vi "Initialise.vi"(4 "Rate (Hz)":dbl=1000.0 format="%0.2f", 6 "WarmupIters":u32=2000, 8 "error in (no error)":errorcluster, 9 "Master Clock":tag, 10 "Tasks Config":T1[](array[typedef]), 11 "PXI in":refnum<class "PXI.lvclass">) -> (0 "error out":errorcluster, 3 "PXI out":refnum<class "PXI.lvclass">)   [LabVIEW 2013, in "PXI.lvclass"]
uses:
  PXI.lvclass
  Task Definition.ctl
  Task Types.ctl
  PXI.lvclass/PXI.ctl
  <vilib>/DAQmx/create/channels.llb/DAQmx Create Channel (AI-Voltage-Basic).vi
  <vilib>/DAQmx/configure/timing.llb/DAQmx Timing (Sample Clock).vi
  <vilib>/DAQmx/create/channels.llb/DAQmx Create Channel (AO-Voltage-Basic).vi
  <vilib>/DAQmx/create/channels.llb/DAQmx Create Channel (DI-Digital Input).vi
  <vilib>/DAQmx/create/channels.llb/DAQmx Create Channel (DO-Digital Output).vi
  <resource>/objmgr/daqmx.rc
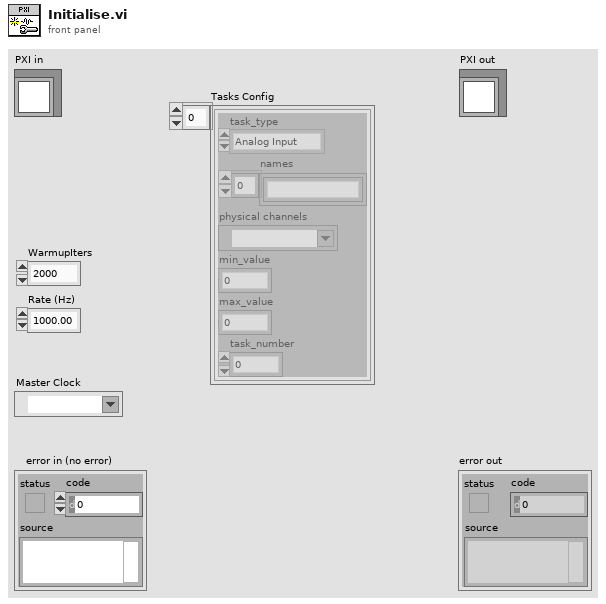
[diagram p1: front panel]
types:
  T1 = typedef "Task Definition.ctl" = cluster{"task_type":T2, "names":string[], "physical channels":tag, "min_value":dbl, "max_value":dbl, "task_number":i32}
  T2 = typedef "Task Types.ctl" = enum16{"Analog Input", "Analog Output", "Digital Input", "Digital Output"}
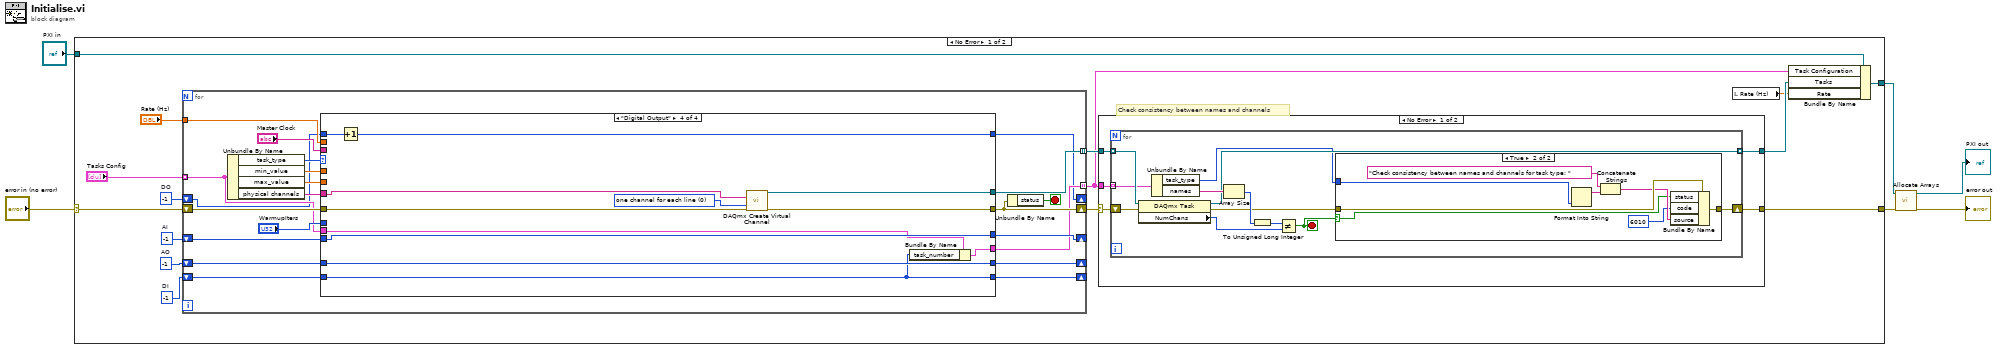
[diagram p0: block diagram]
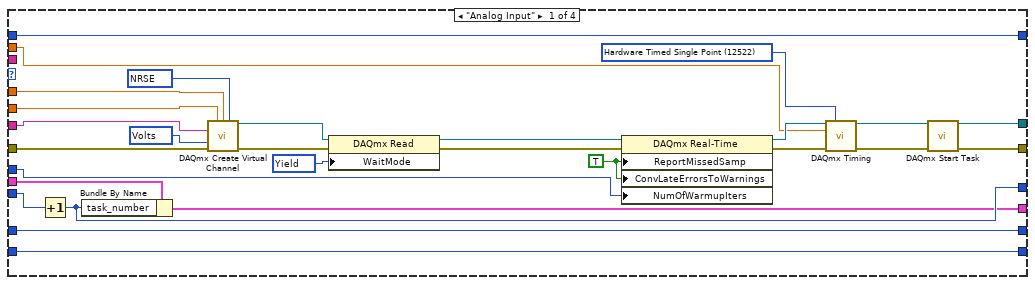
[diagram p4: hidden frame]
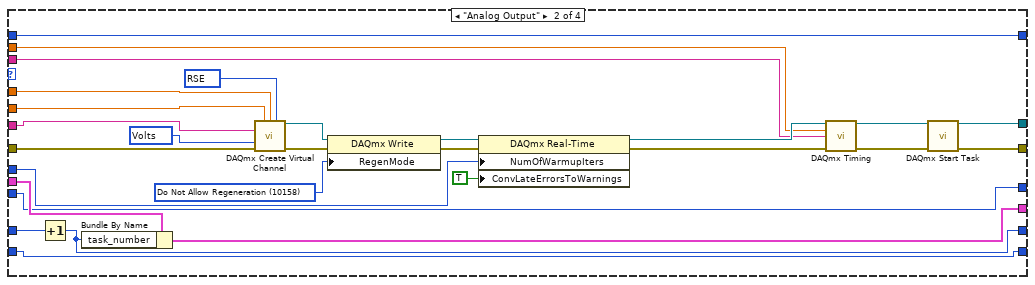
[diagram p5: hidden frame]
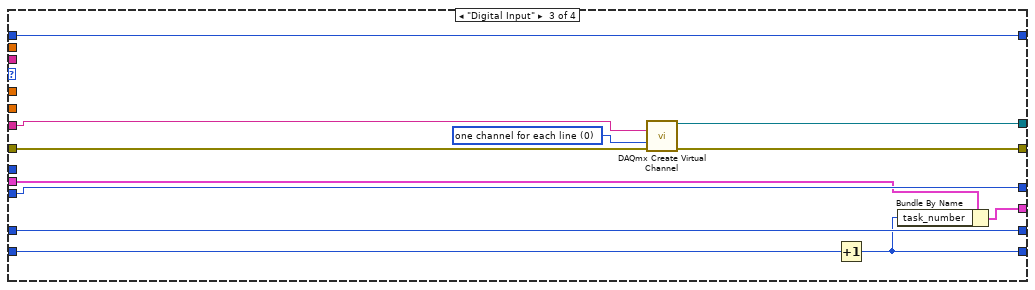
[diagram p6: hidden frame]
diagram:
  n1 = case shown="No Error" "error in (no error)" {
    selector: "error in (no error)" -> [w19 w152]
    tunnel: [w17 w152] -> w3
    tunnel: [w20 w151] -> w4
    tunnel: "PXI in" -> [w21 w151]
    frame No Error {
      w7 = -1  # DO
      w8 = -1  # DI
      w9 = -1  # AO
      w10 = -1  # AI
      # "Check consistency between names and channels"
      n2 = for {
        tunnel: "Tasks Config" -> [w58] mode=indexing
        tunnel: [w65] -> w16 mode=indexing
        shift-right: [w63] -> w18
        shift-left: w19 -> [w64]
        tunnel: "Rate (Hz)" -> [w60]
        tunnel: [w57] -> w11 mode=indexing
        shift-right: [w59] -> _
        shift-left: w10 -> [w56]
        shift-right: [w54] -> _
        shift-left: w9 -> [w55]
        shift-right: [w52] -> _
        shift-left: w8 -> [w53]
        shift-right: [w50] -> _
        shift-left: w7 -> [w51]
        stop <- w62 stop-if-true
        n3 = Unbundle By Name(w58) -> ("task_type"=w61:T2, "min_value"=w69:dbl, "max_value"=w68:dbl, "physical channels"=w67:tag)
        n4 = case shown="\"Digital Output\"" w61 {
          tunnel: w69 -> [w96 w113 _ _]
          tunnel: w68 -> [w95 w112 _ _]
          tunnel: w67 -> [w94 w106 w137 w149]
          tunnel: "WarmupIters" -> [w84 w116 _ _]
          tunnel: "Master Clock" -> [_ w115 _ _]
          tunnel: w60 -> [w83 w114 _ _]
          tunnel: [w80 w109 w136 w148] -> w65
          tunnel: [w79 w108 w135 w147] -> w63
          tunnel: w64 -> [w78 w107 w134 w146]
          tunnel: w56 -> [w77 w101 w133 w145]
          tunnel: [w75 w101 w133 w145] -> w59
          tunnel: w58 -> [w76 w104 w131 w142]
          tunnel: [w74 w103 w130 w143] -> w57
          tunnel: w55 -> [w73 w105 w132 w144]
          tunnel: [w73 w102 w132 w144] -> w54
          tunnel: w53 -> [w72 w100 w129 w139]
          tunnel: [w72 w100 w127 w139] -> w52
          tunnel: w51 -> [w71 w99 w128 w141]
          tunnel: [w71 w99 w128 w140] -> w50
          frame "Analog Input" {
            w85 = TRUE ("ConvLateErrorsToWarnings")
            w88 = 12522 items=["Finite Samples"=10178, "Continuous Samples"=10123, "Hardware Timed Single Point"=12522] ("sample mode")
            w93 = 12525 items=["Wait For Interrupt"=12523, "Poll"=12524, "Yield"=12525, "Sleep"=12547] ("WaitMode")
            w97 = 10348 items=["Volts"=10348, "From Custom Scale"=10065] ("units")
            w98 = 10078 items=["default"=-1, "RSE"=10083, "NRSE"=10078, "Differential"=10106, "Pseudodifferential"=12529] ("input terminal configuration")
            n5 = Increment(x=w77) -> (x+1=w75:i32)
            n6 = Bundle By Name(cluster=w76, "task_number"=w75) -> (w74:T1)
            n7 = call-poly <vilib>:"DAQmx Create Virtual Channel.vi"("maximum value"=w95, "minimum value"=w96, "input terminal configuration"=w98, "physical channels"=w94, "units"=w97, "error in"=w78) -> ("task out"=w87:refnum<k21>, "error out"=w86:errorcluster)  [unwired: 8 in]
            n8 = property class="DAQmx Read"(reference=w87, error in=w86, "WaitMode"=w93) -> (reference out=w91:refnum<k21>, error out=w92:errorcluster)
            n9 = property class="DAQmx Real-Time"(reference=w91, error in=w92, "ReportMissedSamp"=w85, "ConvLateErrorsToWarnings"=w85, "NumOfWarmupIters"=w84) -> (reference out=w89:refnum<k21>, error out=w90:errorcluster)
            n10 = call-poly <vilib>:"DAQmx Timing.vi"("task/channels in"=w89, "sample mode"=w88, "rate"=w83, "error in"=w90) -> ("task out"=w82:refnum<k21>, "error out"=w81:errorcluster)  [unwired: 10 in]
            n11 = call <vilib>:"DAQmx Start Task.vi"("task/channels in"=w82, "error in"=w81) -> ("task out"=w80:refnum<k21>, "error out"=w79:errorcluster)  [unwired: 12 in]
          }
          frame "Analog Output" {
            w123 = 10158 items=["Allow Regeneration"=10097, "Do Not Allow Regeneration"=10158] ("RegenMode")
            w126 = 10083 items=["Default"=-1, "RSE"=10083, "Differential"=10106, "Pseudodifferential"=12529] ("output terminal configuration")
            w125 = 10348 items=["Volts"=10348, "From Custom Scale"=10065] ("units")
            n12 = Increment(x=w105) -> (x+1=w102:i32)
            n13 = Bundle By Name(cluster=w104, "task_number"=w102) -> (w103:T1)
            n14 = call-poly <vilib>:"DAQmx Create Virtual Channel.vi"("maximum value"=w112, "minimum value"=w113, "output terminal configuration"=w126, "physical channels"=w106, "units"=w125, "error in"=w107) -> ("task out"=w122:refnum<k21>, "error out"=w121:errorcluster)  [unwired: 8 in]
            n15 = property class="DAQmx Write"(reference=w122, error in=w121, "RegenMode"=w123) -> (reference out=w120:refnum<k21>, error out=w119:errorcluster)
            n16 = property class="DAQmx Real-Time"(reference=w120, error in=w119, "NumOfWarmupIters"=w116, "ConvLateErrorsToWarnings"=TRUE ("ReportMissedSamp")) -> (reference out=w118:refnum<k21>, error out=w117:errorcluster)
            n17 = call-poly <vilib>:"DAQmx Timing.vi"("task/channels in"=w118, "rate"=w114, "source"=w115, "error in"=w117) -> ("task out"=w111:refnum<k21>, "error out"=w110:errorcluster)  [unwired: 10 in]
            n18 = call <vilib>:"DAQmx Start Task.vi"("task/channels in"=w111, "error in"=w110) -> ("task out"=w109:refnum<k21>, "error out"=w108:errorcluster)  [unwired: 12 in]
          }
          frame "Digital Input" {
            w138 = 0 items=["one channel for each line", "one channel for all lines"] ("line grouping")
            n19 = call-poly <vilib>:"DAQmx Create Virtual Channel.vi"("lines"=w137, "line grouping"=w138, "error in"=w134) -> ("task out"=w136:refnum<k21>, "error out"=w135:errorcluster)  [unwired: 11 in]
            n20 = Increment(x=w129) -> (x+1=w127:i32)
            n21 = Bundle By Name(cluster=w131, "task_number"=w127) -> (w130:T1)
          }
          frame "Digital Output" {
            w150 = 0 items=["one channel for each line", "one channel for all lines"] ("line grouping")
            n22 = Increment(x=w141) -> (x+1=w140:i32)
            n23 = call-poly <vilib>:"DAQmx Create Virtual Channel.vi"("lines"=w149, "line grouping"=w150, "error in"=w146) -> ("task out"=w148:refnum<k21>, "error out"=w147:errorcluster)  [unwired: 11 in]
            n24 = Bundle By Name(cluster=w142, "task_number"=w139) -> (w143:T1)
          }
        }
        n25 = Unbundle By Name(w63) -> ("status"=w62:bool)
      }
      n26 = case shown="No Error" w18 {
        selector: w18 -> [w24 w49]
        tunnel: [w22 w49] -> w17
        tunnel: w16 -> [w25 w48]
        tunnel: w11 -> [w26 _]
        tunnel: [w23 w48] -> w14
        frame No Error {
          n27 = for {
            tunnel: w26 -> [w36] mode=indexing
            tunnel: w25 -> [w38] mode=indexing
            tunnel: [w31] -> w23 mode=indexing
            shift-right: [w28] -> w22
            shift-left: w24 -> [w37]
            stop <- w30 stop-if-true
            n28 = property class="DAQmx Task"(reference=w38, error in=w37) -> (reference out=w31:refnum<k21>, error out=w29:errorcluster, "NumChans"=w34:u32)
            n29 = Unbundle By Name(w36) -> ("task_type"=w27:T2, "names"=w35:string[])
            n30 = Array Size(array=w35) -> (size(s)=w33:i32)
            n31 = To Unsigned Long Integer(number=w33) -> (unsigned 32bit integer=w32:u32)
            n32 = Not Equal?(x=w32, y=w34) -> (x != y?=w30:bool)
            n33 = case shown="True" w30 {
              selector: w30 -> [_ w40]
              tunnel: w29 -> [w39 w47]
              tunnel: [w39 w46] -> w28
              tunnel: w27 -> [_ w45]
              frame False {
              }
              frame True {
                n34 = Format Into String(w45) -> (resulting string=w44:string)  [unwired: 3 in, 1 out]
                n35 = Concatenate Strings("Check consistency between names and channels for task type: " ("source"), w44) -> (w42:string)
                n36 = Bundle By Name(cluster=w47, "status"=w40, "code"=6010, "source"=w42) -> (w46:errorcluster)
              }
            }
          }
        }
        frame Error {
        }
      }
      n37 = local read "Rate (Hz)"() -> (w12:dbl)
      n38 = Bundle By Name(cluster=w21, "Task Configuration"=w11, "Tasks"=w14, "Rate"=w12) -> (w20:refnum<class "PXI.lvclass">)
    }
    frame Error {
    }
  }
  n39 = call "Allocate Arrays.vi"("error in (no error)"=w3, "PXI in"=w4) -> ("error out"=→"error out":errorcluster, "PXI out"=→"PXI out":refnum<class "PXI.lvclass">)  [unwired: 8 in]
